vi "Start Sync.vi"(8 "error in (no error)":errorcluster, 11 "gRPC Server in":refnum<class "stream.lvclass">) -> (0 "error out":errorcluster, 3 "gRPC Server out":refnum<class "stream.lvclass">)   [LabVIEW 2021, in "streamtest_server.lvlib" / "stream.lvclass"]
uses:
  stream.lvclass
  stream.lvclass/stream.ctl
  RPC Messages/streamtest_StreamData.ctl
  streamtest_server.lvlib
panel:
  out "error out 2":errorcluster
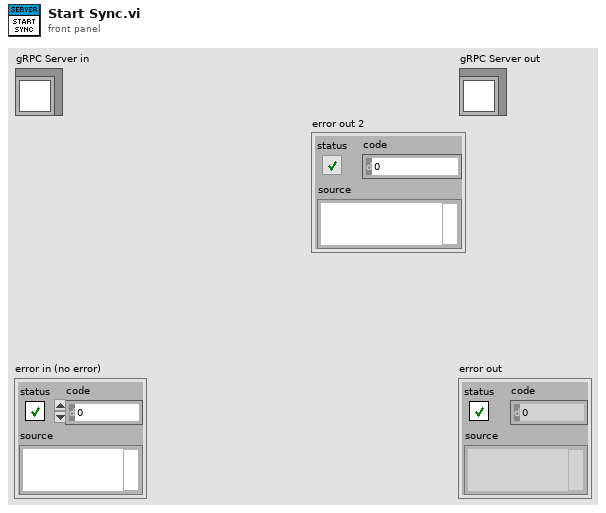
[diagram p1: front panel]
types:
  T1 = typedef "streamtest_server.lvlib/streamtest_StreamData.ctl" = cluster{"stream_data":u8[]}
  T2 = typedef "streamtest_server.lvlib/stream.lvclass/Server Internal UEs.ctl" = cluster{"stream Send Internal UE":refnum<user-event>}
  T3 = typedef "streamtest_server.lvlib/stream.lvclass/Server gRPC UEs.ctl" = cluster{"stream Send gRPC UE":refnum<user-event>}
  T4 = typedef "grpc-lvsupport-release.lvlib/grpcId.ctl" = u64
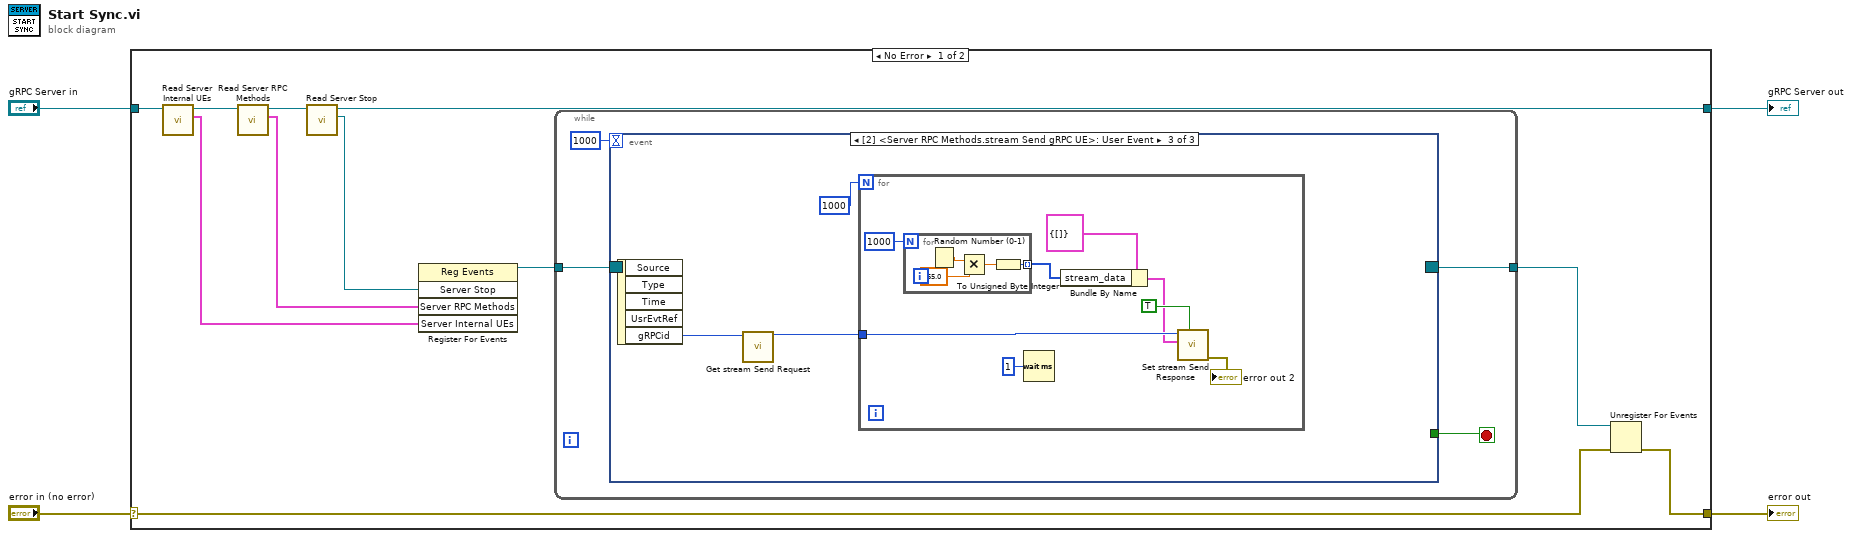
[diagram p0: block diagram]
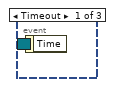
[diagram p2: hidden frame]
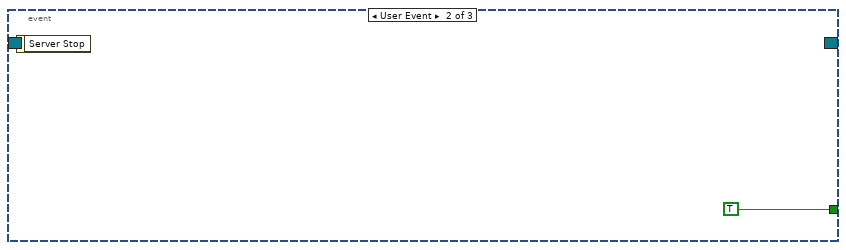
[diagram p3: hidden frame]
diagram:
  n1 = case shown="No Error" "error in (no error)" {
    selector: "error in (no error)" -> [w9 w37]
    tunnel: [w8 w37] -> w3
    tunnel: [w6 w36] -> w1
    tunnel: "gRPC Server in" -> [w15 w36]
    frame No Error {
      n2 = call "Read Server Internal UEs.vi"("SignalGeneratorService in"=w15) -> ("Server Internal UEs"=w13:T2, "SignalGeneratorService out"=w14:refnum<class "stream.lvclass">)  [unwired: 8 in, 1 out]
      n3 = call "Read Server RPC Methods.vi"("SignalGeneratorService in"=w14) -> ("Server RPC Methods"=w7:T3, "SignalGeneratorService out"=w12:refnum<class "stream.lvclass">)  [unwired: 8 in, 1 out]
      n4 = call-dynamic "Read Server Stop.vi"("iService in"=w12) -> ("Server Stop"=w5:refnum<user-event>, "iService out"=w6:refnum<class "stream.lvclass">)  [unwired: 8 in, 1 out]
      n5 = register-events(w5, w7, w13) -> (reference out=w11:refnum<event-registration>)  [unwired: 2 in, 1 out]
      n6 = while {
        tunnel: w11 -> [w19]
        tunnel: [w17] -> w10
        stop <- w18 stop-if-true
        n7 = event "RPC Methods Event Structure" shown="[2] <Server RPC Methods.stream Send gRPC UE>: User Event" {
          selector: w19 -> [_ _ _]
          dyn-events: [_ _ _] -> w17
          timeout: 1000 -> [_ _ _]
          tunnel: [_ TRUE _] -> w18
          event Timeout {
            n8 = event-data() -> ()  [unwired: 1 in, 1 out]
          }
          event User Event {
            n9 = event-data() -> ()  [unwired: 1 in, 1 out]
          }
          event User Event {
            n10 = event-data() -> ("gRPCid"=w23:T4)  [unwired: 1 in, 4 out]
            n11 = call "Get stream Send Request.vi"("gRPCid"=w23) -> ("gRPCid out"=w22:T4)  [unwired: 8 in, 2 out]
            n12 = for {
              N: 1000 -> [_]
              tunnel: w22 -> [w31]
              n13 = for {
                N: 1000 -> [_]
                tunnel: [w32] -> w27 mode=indexing
                n14 = Random Number (0-1)() -> (number: 0 to 1=w35:dbl)
                n15 = Multiply(x=w35, y=255.0) -> (x*y=w33:dbl)
                n16 = To Unsigned Byte Integer(number=w33) -> (unsigned 8bit integer=w32:u8)
              }
              n17 = Wait (ms)(milliseconds to wait=u32 1) -> ()  [unwired: 1 out]
              n18 = Bundle By Name(cluster=T1 {"stream_data"=[]} ("Message Data"), "stream_data"=w27) -> (w26:T1)
              n19 = call "Set stream Send Response.vi"("Streaming? (F)"=TRUE, "Message Data"=w26, "gRPCid in"=w31) -> ("error out"=→"error out 2":errorcluster)  [unwired: 8 in]
            }
          }
        }
      }
      n20 = Unregister For Events(event registration refnum=w10, error in=w9) -> (error out=w8:errorcluster)
    }
    frame Error {
    }
  }
  "error out" <- w3
  "gRPC Server out" <- w1
